vi "UDP Multicast Receiver Test.vi"() -> ()   [LabVIEW 2020]
uses:
  <vilib>/Utility/tcp.llb/UDP Multicast Read-Only Open.vi
panel:
  out "Array":string[](array[string])
  out "data out 2":string
  out "data out":string
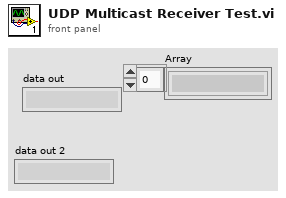
[diagram p1: front panel]
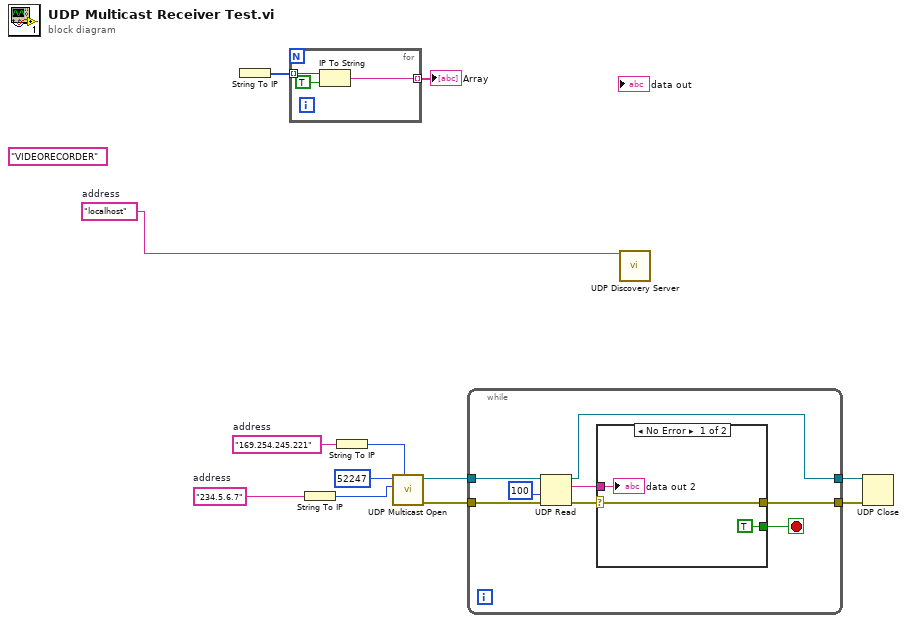
[diagram p0: block diagram]
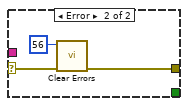
[diagram p2: hidden frame]
diagram:
  (unwired) "VIDEORECORDER"
  w9 = "234.5.6.7"  # address
  w11 = "169.254.245.221"  # address
  w1 = "localhost"  # address
  n1 = String To IP() -> (0:w3:u32[])  [unwired: 1 in]
  n2 = for {
    tunnel: w3 -> [w15] mode=indexing
    tunnel: [w14] -> w2 mode=indexing
    n3 = IP To String(1:TRUE ("dot notation? (F)"), 2:w15) -> (0:w14:string)
  }
  "Array" <- w2
  n4 = String To IP(1:w9) -> (0:w8:u32)
  n5 = String To IP(1:w11) -> (0:w10:u32)
  n6 = call-poly <vilib>:"UDP Multicast Open.vi"("net address"=w10, "multicast addr"=w8, "port"=u16 52247) -> ("error out"=w6:errorcluster, "connection ID"=w7:refnum<k16>)  [unwired: 6 in, 1 out]
  n7 = while {
    tunnel: w7 -> [w22]
    tunnel: w6 -> [w21]
    tunnel: [w19] -> w5
    tunnel: [w18] -> w4
    stop <- w16 stop-if-true
    n8 = UDP Read(connection ID=w22, timeout ms (25000)=100, 8:w21) -> (data out=w17:string, error out=w20:errorcluster, 3:w18:refnum<k16>)  [unwired: 3 out]
    n9 = case shown="No Error" w20 {
      selector: w20 -> [w25 w29]
      tunnel: [w25 w27] -> w19
      tunnel: w17 -> [w26 _]
      tunnel: [TRUE _] -> w16
      frame No Error {
        "data out 2" <- w26
      }
      frame Error {
        n10 = call <vilib>:"Clear Errors.vi"("error in (no error)"=w29, "specific error code to clear (0: all)"=56) -> ("error out"=w27:errorcluster)  [unwired: 4 in, 1 out]
      }
    }
  }
  n11 = call "UDP Discovery Server.vi"("Name"=w1) -> ()  [unwired: 14 in, 1 out]
  n12 = UDP Close(connection ID=w4, 8:w5) -> ()  [unwired: 2 out]
